vi "selectPara.vi"() -> ()   [LabVIEW 2010]
panel:
  in  "重置":bool
  in  "A-21":bool
  in  "A-20":bool
  in  "A-19":bool
  in  "A-18":bool
  in  "A-17":bool
  in  "A-16":bool
  in  "A-15":bool
  in  "A-14":bool
  in  "A-13":bool
  in  "A-12":bool
  in  "A-11":bool
  in  "A-10":bool
  in  "A-9":bool
  in  "A-8":bool
  in  "A-7":bool
  in  "A-6":bool
  in  "A-5":bool
  in  "A-4":bool
  in  "A-3":bool
  in  "A-2":bool
  in  "A-1":bool
  in  "V-21":bool
  in  "电网频率":bool
  in  "取消":bool
  in  "确定":bool
  in  "V-20":bool
  in  "V-19":bool
  in  "V-18":bool
  in  "V-17":bool
  in  "V-16":bool
  in  "V-15":bool
  in  "V-14":bool
  in  "V-13":bool
  in  "V-12":bool
  in  "V-11":bool
  in  "V-10":bool
  in  "V-9":bool
  in  "V-8":bool
  in  "V-7":bool
  in  "V-6":bool
  in  "V-5":bool
  in  "V-4":bool
  in  "V-3":bool
  in  "V-2":bool
  in  "V-1":bool
  in  "反向有功基波电能":bool
  in  "正向有功基波电能":bool
  in  "反向有功谐波电能":bool
  in  "正向有功谐波电能":bool
  in  "生产日期":bool
  in  "协议版本号":bool
  in  "电表地址":bool
  in  "反向视在电能":bool
  in  "正向视在电能":bool
  in  "电表型号":bool
  in  "额定电流":bool
  in  "额定电压":bool
  in  "反向有功电能":bool
  in  "正向有功电能":bool
  in  "表内温度":bool
  in  "零线电流":bool
  in  "A相电流谐波含量数据块":bool
  in  "A相电压谐波含量数据块":bool
  in  "A相电流":bool
  in  "A相电流波形失真度":bool
  in  "A相电压波形失真度":bool
  in  "A相相角":bool
  in  "A相功率因数":bool
  in  "A相瞬时视在功率":bool
  in  "A相瞬时无功功率":bool
  in  "A相瞬时有功功率":bool
  in  "A相电压":bool
  out "Exit":bool=TRUE
  # "A相电能参数选择"
  # "A相电压谐波含量"
  # "A相电流谐波含量"
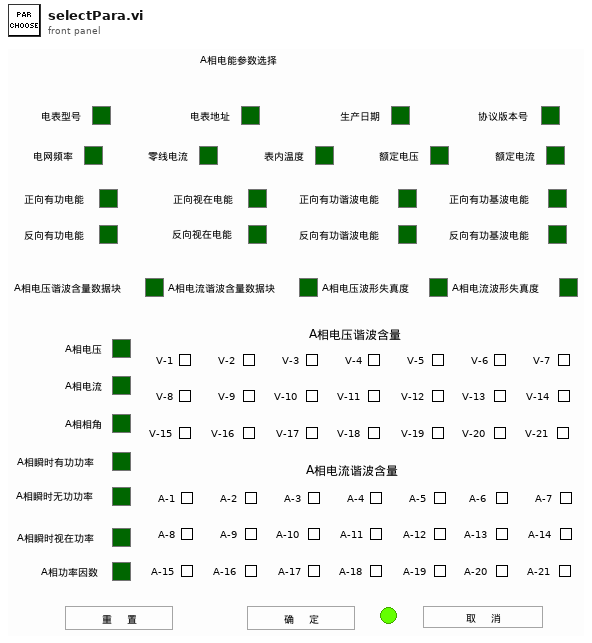
[diagram p1: front panel]
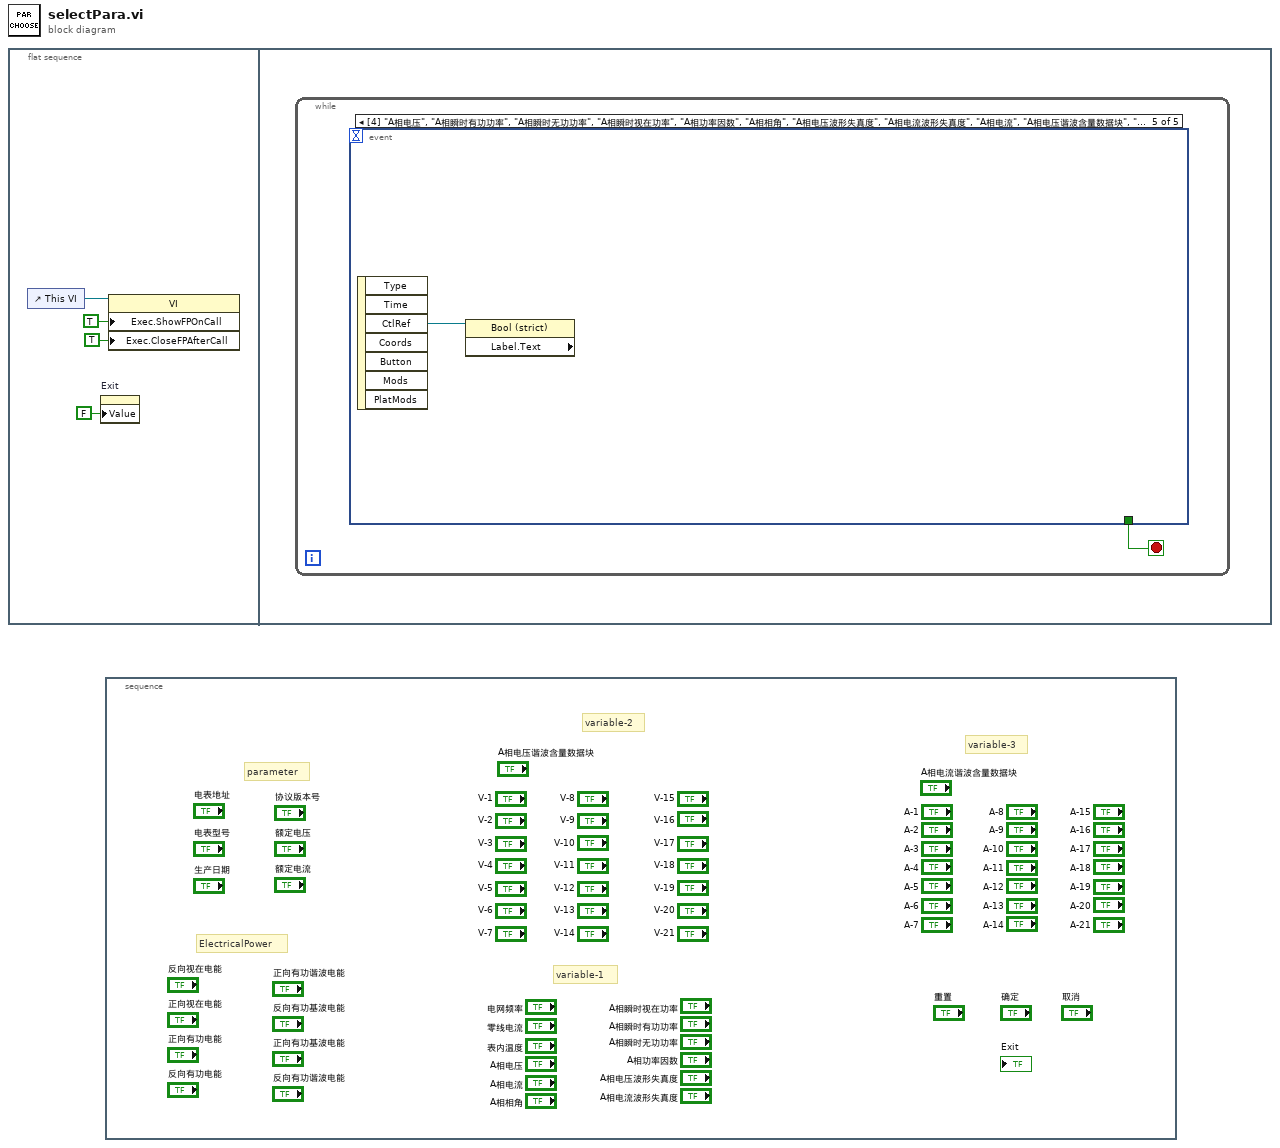
[diagram p0: block diagram]
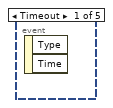
[diagram p2: hidden frame]
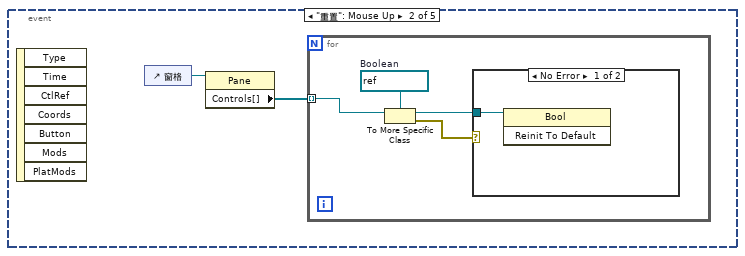
[diagram p3: hidden frame]
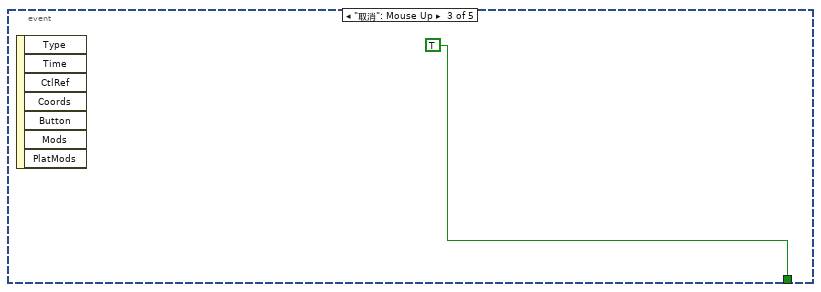
[diagram p5: hidden frame]
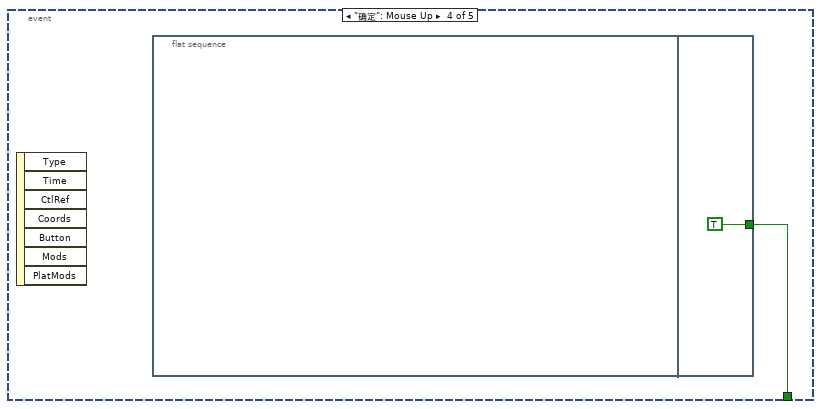
[diagram p6: hidden frame]
diagram:
  n1 = flat-sequence {
    frame #0 {
      n2 = control-ref of="This VI"() -> (w4:refnum<vi>)
      n3 = property on="Exit" class="Bool (strict)"("Value"=FALSE ("Exit")) -> ()  [unwired: 2 in, 2 out]
      n4 = property class="VI"(reference=w4, "Exec.ShowFPOnCall"=TRUE ("Execution:Show Front Panel On Call"), "Exec.CloseFPAfterCall"=TRUE ("Execution:Close After Call")) -> ()  [unwired: 1 in, 2 out]
    }
    frame #1 {
      n5 = while {
        stop <- w5 stop-if-true
        n6 = event shown="[4] \"A相电压\", \"A相瞬时有功功率\", \"A相瞬时无功功率\", \"A相瞬时视在功率\", \"A相功率因数\", \"A相相角\", \"A相电压波形失真度\", \"A相电流波形失真度\", \"A相电流\", \"A相电压谐波含量数据块\", \"A相电流谐波含量数据块\", \"零线电流\", \"表内温度\", \"正向有功电能\", \"反向有功电能\", \"额定电压\", \"额定电流\", \"电表型号\", \"正向视在电能\", \"反向视在电能\", \"电表地址\", \"协议版本号\": Mouse Up" {
          selector: _ -> [_ _ _ _ _]
          dyn-events: _ -> [_ _ _ _ _]
          timeout: _ -> [_ _ _ _ _]
          tunnel: [_ _ TRUE ("Exit") w14 _] -> w5
          event Timeout {
            n7 = event-data() -> ()  [unwired: 1 in, 2 out]
          }
          event "重置": Mouse Up {
            n8 = event-data() -> ()  [unwired: 1 in, 7 out]
            n9 = control-ref of="窗格"() -> (w6:refnum<vi>)
            n10 = property class="Pane"(reference=w6) -> ("Controls[]"=w7:refnum<vi>[])  [unwired: 1 in, 2 out]
            n11 = for {
              tunnel: w7 -> [w8] mode=indexing
              w11 = refnum<vi> refnum  # Boolean
              n12 = To More Specific Class(target class=w11, reference=w8) -> (specific class reference=w9:refnum<vi>, error out=w10:errorcluster)  [unwired: 1 in]
              n13 = case shown="No Error" w10 {
                tunnel: w9 -> [w12 _]
                frame No Error {
                  n14 = invoke class="Bool" method="Reinit To Default"(reference=w12) -> ()  [unwired: 2 in, 3 out]
                }
                frame Error {
                }
              }
            }
          }
          event "取消": Mouse Up {
            n15 = event-data() -> ()  [unwired: 1 in, 7 out]
          }
          event "确定": Mouse Up {
            n16 = event-data() -> ()  [unwired: 1 in, 7 out]
            n17 = flat-sequence {
              tunnel: [TRUE ("Exit")] -> w14
              frame #0 {
              }
              frame #1 {
              }
            }
          }
          event "A相电压", "A相瞬时有功功率", "A相瞬时无功功率", "A相瞬时视在功率", "A相功率因数", "A相相角", "A相电压波形失真度", "A相电流波形失真度", "A相电流", "A相电压谐波含量数据块", "A相电流谐波含量数据块", "零线电流", "表内温度", "正向有功电能", "反向有功电能", "额定电压", "额定电流", "电表型号", "正向视在电能", "反向视在电能", "电表地址", "协议版本号": Mouse Up {
            n18 = event-data() -> ("CtlRef"=w16:refnum<vi>)  [unwired: 1 in, 6 out]
            n19 = property class="Bool (strict)" props=["Label", "Text"](reference=w16) -> ()  [unwired: 1 in, 3 out]
          }
        }
      }
    }
  }
  n20 = stacked-sequence {
    frame #0 {
      # "ElectricalPower"
      # "variable-3"
      # "variable-2"
      # "variable-1"
      # "parameter"
    }
  }
